vi "(SubVI) Pull DNA_YCC.vi"(0 "task/channels in":refnum<k21>, 1 "Filter type":T1(ring), 2 "Avg points":i32, 3 "Real initial position (um)":dbl format="%0.5f", 5 "Record?":bool, 7 "T=X\nF=Y":bool, 9 "Toward  ?\nT=+, F=-":bool, 11 "error in":errorcluster, 12 "Record scan rate  (um/s)":dbl=2.0 format="%.3f", 13 "range  (um)":dbl=2.0 min=0.0 max=100.0 step=0.5 format="%.3f", 14 "Sampling rate":dbl=20000.0 format="%0.2f") -> (4 "task out":refnum<k21>, 6 "Raw Stage Array":dbl[](array[numeric]), 8 "Filtered Stage Array":dbl[](array[numeric]) format="%0.2f", 10 "Filtered QPD Array":dbl[](array[numeric]) format="%0.2f", 15 "error out":errorcluster)   [LabVIEW 2014]
uses:
  <vilib>/DAQmx/read.llb/DAQmx Read (Analog 1D DBL 1Chan NSamp).vi
panel:
  in  "no Record scan rate  (um/s)":dbl=2.0
  out "scan rate  (um/s)":dbl
  out "True rate?":bool
  out "axis":u32=1
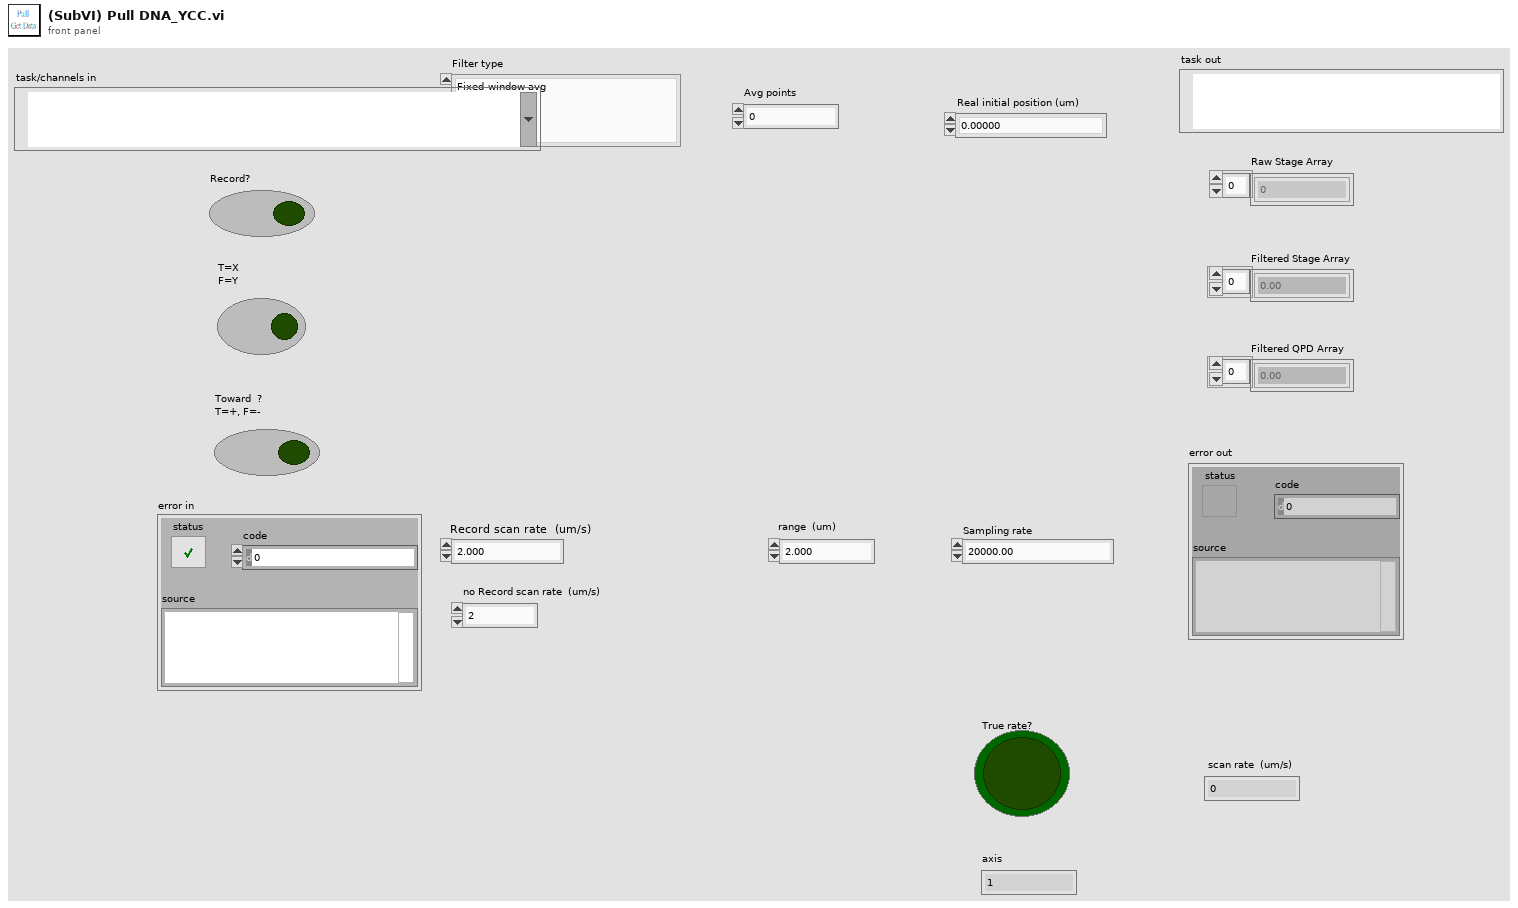
[diagram p1: front panel]
types:
  T1 = enum16{"Fixed-window avg", "Moving-window avg", "S-G filter", "Median filter"}
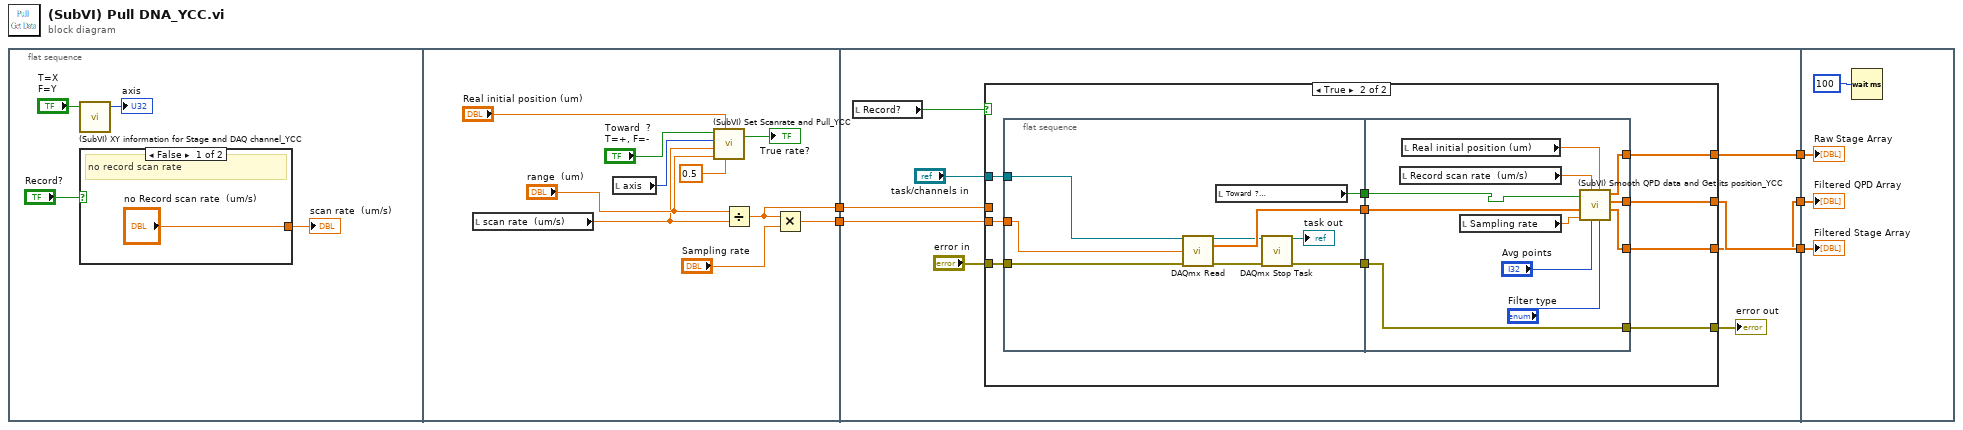
[diagram p0: block diagram]
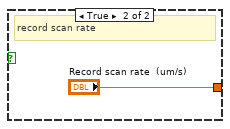
[diagram p2: hidden frame]
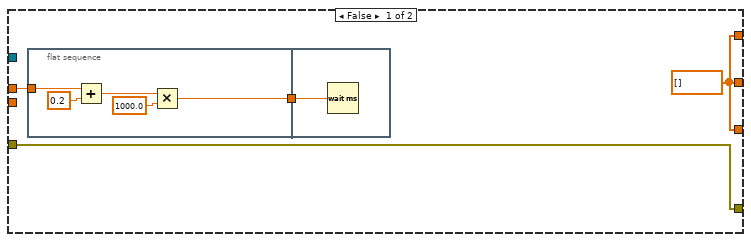
[diagram p3: hidden frame]
diagram:
  n1 = flat-sequence {
    tunnel: [w18] -> w5
    tunnel: [w12] -> w4
    tunnel: w5 -> [w30]
    tunnel: w4 -> [w26]
    tunnel: [w25] -> w3
    tunnel: [w23] -> w2
    tunnel: [w22] -> w1
    tunnel: w3 -> [w74]
    tunnel: w2 -> [w73]
    tunnel: w1 -> [w72]
    frame #0 {
      n2 = call "(SubVI) XY information for Stage and DAQ channel_YCC.vi"("T=X\nF=Y"="T=X\nF=Y") -> ("Axis"=→"axis":i32)  [unwired: 3 in, 1 out]
      n3 = case shown="False" "Record?" {
        tunnel: ["no Record scan rate  (um/s)" "Record scan rate  (um/s)"] -> w6
        frame False {
          # "no record scan rate"
        }
        frame True {
          # "record scan rate"
        }
      }
      "scan rate  (um/s)" <- w6
    }
    frame #1 {
      n4 = local read "scan rate  (um/s)"() -> (w13:dbl)
      n5 = local read "axis"() -> (w19:u32)
      n6 = call "(SubVI) Set Scanrate and Pull_YCC.vi"("waiting time per point (ms)\nrange from 5ms to 0.167 ms"=0.5 ("waiting time per point (ms)\nrange from 5ms to 0.167 ms"), "Start From  (um)"="Real initial position (um)", "range  (um)"="range  (um)", "scan rate  (um/s)"=w13, "axis"=w19, "toward+ ?\nT=+, F=-"="Toward  ?\nT=+, F=-") -> ("True rate?"=→"True rate?":bool)  [unwired: 1 out]
      n7 = Divide(x="range  (um)", y=w13) -> (x/y=w12:dbl)
      n8 = Multiply(x=w12, y="Sampling rate") -> (x*y=w18:dbl)
    }
    frame #2 {
      n9 = local read "Record?"() -> (w29:bool)
      n10 = case shown="True" w29 {
        tunnel: "error in" -> [w34 w50]
        tunnel: w30 -> [_ w49]
        tunnel: [w34 w48] -> w27
        tunnel: w26 -> [w32 _]
        tunnel: [w33 w44] -> w25
        tunnel: [w33 w43] -> w22
        tunnel: [w33 w42] -> w23
        tunnel: "task/channels in" -> [_ w41]
        frame False {
          w33 = dbl[] [] ("data")
          n11 = flat-sequence {
            tunnel: w32 -> [w37]
            tunnel: [w38] -> w31
            tunnel: w31 -> [w40]
            frame #0 {
              n12 = Add(x=w37, y=0.2) -> (x+y=w35:dbl)
              n13 = Multiply(x=w35, y=1000.0) -> (x*y=w38:dbl)
            }
            frame #1 {
              n14 = Wait (ms)(milliseconds to wait=w40) -> ()  [unwired: 1 out]
            }
          }
        }
        frame True {
          n15 = flat-sequence {
            tunnel: w50 -> [w59]
            tunnel: w49 -> [w58]
            tunnel: [w57] -> w47
            tunnel: [w56] -> w46
            tunnel: [w52] -> w45
            tunnel: w41 -> [w51]
            tunnel: [w70] -> w48
            tunnel: w47 -> [w60]
            tunnel: w46 -> [w64]
            tunnel: w45 -> [w70]
            tunnel: [w63] -> w44
            tunnel: [w62] -> w43
            tunnel: [w61] -> w42
            frame #0 {
              n16 = call-poly <vilib>:"DAQmx Read.vi"("task/channels in"=w51, "number of samples per channel"=w58, "error in"=w59) -> ("task out"=w55:refnum<k21>, "data"=w56:dbl[], "error out"=w54:errorcluster)  [unwired: 10 in]
              n17 = local read "Toward  ?\nT=+, F=-"() -> (w57:bool)
              n18 = call <vilib>:"DAQmx Stop Task.vi"("task/channels in"=w55, "error in"=w54) -> ("task out"=→"task out":refnum<k21>, "error out"=w52:errorcluster)  [unwired: 12 in]
            }
            frame #1 {
              n19 = local read "Record scan rate  (um/s)"() -> (w65:dbl)
              n20 = local read "Real initial position (um)"() -> (w69:dbl)
              n21 = local read "Sampling rate"() -> (w67:dbl)
              n22 = call "(SubVI) Smooth QPD data and Get its position_YCC.vi"("Filter type"="Filter type", "Initial position (um)"=w69, "Avg points"="Avg points", "scan rate  (um/s)"=w65, "Sampling rate (Hz)"=w67, "QPD data"=w64, "Direction\nT=+ \nF=-"=w60) -> ("Filtered QPD data"=w62:dbl[], "Filtered Stage Array"=w61:dbl[], "Raw Stage Array"=w63:dbl[])  [unwired: 2 in]
            }
          }
        }
      }
      "error out" <- w27
    }
    frame #3 {
      n23 = Wait (ms)(milliseconds to wait=u32 100) -> ()  [unwired: 1 out]
      "Raw Stage Array" <- w74
      "Filtered Stage Array" <- w73
      "Filtered QPD Array" <- w72
    }
  }
